vi "REPORT_GEAR_rows_style_pdf.vi"(11 "REPORT_GEAR_all_info":T1) -> (3 "Row  [ ]":T4)   [LabVIEW 2020]
uses:
  <vilib>/Exaprom PDF/Controls/Table Controls/Table Appearance and Font Row [ ].ctl
  <vilib>/Exaprom PDF/Controls/Table Controls/One Row Appearance.ctl
  <vilib>/Exaprom PDF/Controls/Table Controls/Row from to.ctl
  <vilib>/Exaprom PDF/Controls/Table Controls/Cell, Alignment, LS and Font - hide Vmerge.ctl
  <vilib>/Exaprom PDF/Controls/Table Controls/Cell Type, Alignment and LS.ctl
  <vilib>/Exaprom PDF/Controls/Table Controls/Cell Alignment 20px.ctl
  <vilib>/Exaprom PDF/Controls/Table Controls/Text vertical arrangement.ctl
  <vilib>/Exaprom PDF/Controls/Text Controls/Line spacing.ctl
  <vilib>/Exaprom PDF/Controls/Table Controls/Cell Appearance.ctl
  <vilib>/Exaprom PDF/Controls/Table Controls/Cell Border 20 px.ctl
  <vilib>/Exaprom PDF/Controls/Table Controls/Merge Horizontal.ctl
  <vilib>/Exaprom PDF/Controls/Table Controls/Merge Vertical.ctl
  <vilib>/Exaprom PDF/Controls/Font Controls/Font complete cluster.ctl
  <vilib>/Exaprom PDF/Controls/Font Controls/Font size.ctl
  <vilib>/Exaprom PDF/Controls/Font Controls/Font color.ctl
  <vilib>/Exaprom PDF/Controls/Font Controls/Type and encoding.ctl
  <vilib>/Exaprom PDF/Controls/Text Controls/Unicode/Type and run direction.ctl
  typedef/REPORT_GEAR_all_info.ctl
  typedef/REPORT_GEAR_header_data_display.ctl
  typedef/REPORT_GEAR_statuses.ctl
panel:
  # "GEAR INFO SUMMARY"
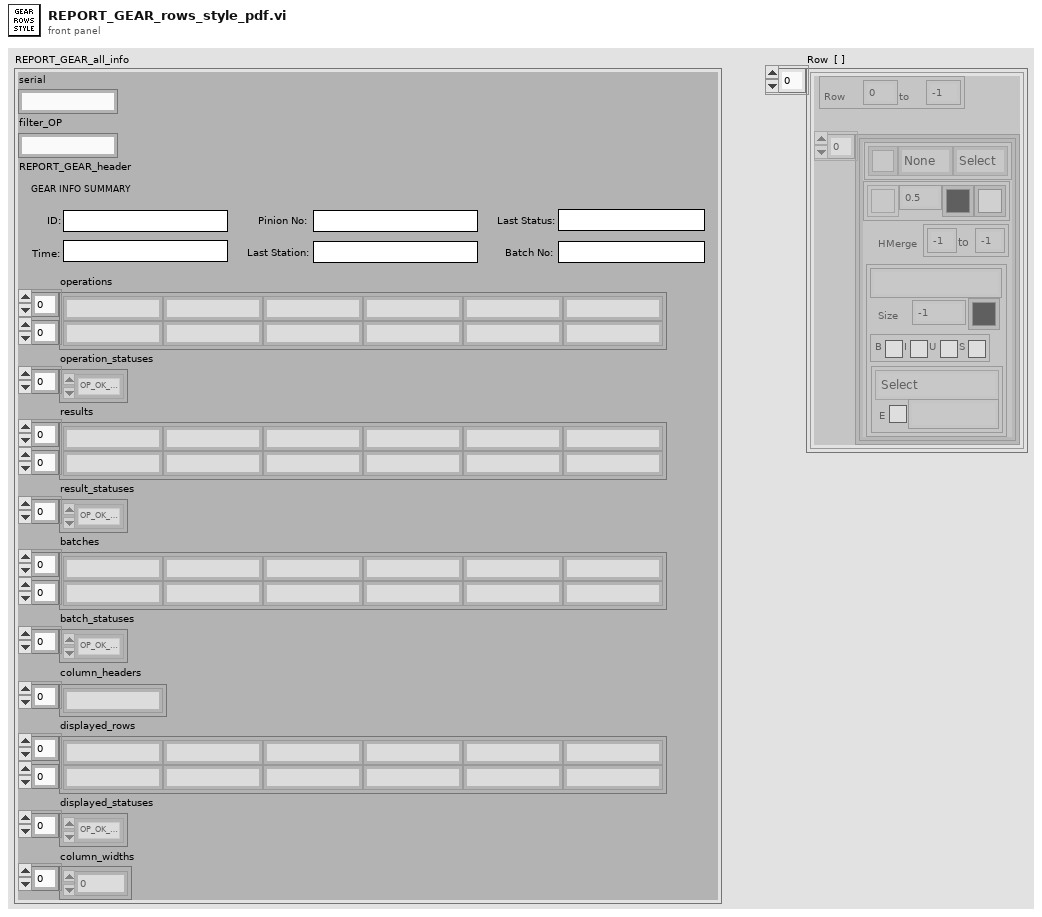
[diagram p1: front panel]
types:
  T1 = typedef "REPORT_GEAR_all_info.ctl" = cluster{"serial":string, "filter_OP":string, "REPORT_GEAR_header":T2, "operations":string[][], "operation_statuses":T3[], "results":string[][], "result_statuses":T3[], "batches":string[][], "batch_statuses":T3[], "column_headers":string[], "displayed_rows":string[][], "displayed_statuses":T3[], "column_widths":i16[]}
  T2 = typedef "REPORT_GEAR_header_data_display.ctl" = cluster{"ID":string, "creation_time":string, "last_station":string, "last_status":string, "pinion_serial":string, "batch_code":string}
  T3 = typedef "REPORT_GEAR_statuses.ctl" = enum16{"OP_OK_hide", "OP_OK_show", "OP_NOK_hide", "OP_NOK_show", "OP_interrupted_hide", "OP_interrupted_show", "OP_in_operation_hide", "OP_in_operation_show", "OP_unexpected_hide", "OP_unexpected_show", "RE_REAL_OK", "RE_REAL_NOK", "RE_STRING", "RE_sub_header", "RE_no_data", "RE_unexpected", "BA_sub_header", "BA_data", "BA_no_data", "AUDIT_RESULT_OK", "AUDIT_RESULT_NOK", "AUDIT_RESULT_UNEXPECTED"}
  T4 = typedef "Table Appearance and Font Row [ ].ctl" = T5[]
  T5 = typedef "One Row Appearance.ctl" = cluster{"Row":T6, "Cell [ ]":T7[]}
  T6 = typedef "Row from to.ctl" = cluster{"From #":i16, "to #":i16}
  T7 = typedef "Cell, Alignment, LS and Font - hide Vmerge.ctl" = cluster{"Text":T8, "Cell Appearance":T12, "HMerge":T14, "VMerge":T15, "Font":T16}
  T8 = typedef "Cell Type, Alignment and LS.ctl" = cluster{"Cell Alignment":T9, "Text rotation":T10, "Line spacing":T11}
  T9 = typedef "Cell Alignment 20px.ctl" = u16
  T10 = typedef "Text vertical arrangement.ctl" = enum16{"None", "Clockwise", "Counterclockwise"}
  T11 = typedef "Line spacing.ctl" = enum16{"Select", "1.0", "1.5", "2.0"}
  T12 = typedef "Cell Appearance.ctl" = cluster{"Border":T13, "Thickness":sgl, "Color":u32, "BG":u32}
  T13 = typedef "Cell Border 20 px.ctl" = u16
  T14 = typedef "Merge Horizontal.ctl" = cluster{"From":i8, "to":i8}
  T15 = typedef "Merge Vertical.ctl" = cluster{"From":i8, "to":i8}
  T16 = typedef "Font complete cluster.ctl" = cluster{"Name":string, "Size":T17, "Color":T18, "Style":cluster{"Bold":bool, "Italic":bool, "Underline":bool, "Strikeout":bool}, "Type":T19}
  T17 = typedef "Font size.ctl" = sgl
  T18 = typedef "Font color.ctl" = u32
  T19 = typedef "Type and encoding.ctl" = cluster{"Type&direction":T20, "Embedded":bool, "Encoding":string}
  T20 = typedef "Type and run direction.ctl" = enum16{"Select", "ASCII", "UTF-16", "UTF-16 (default)", "UTF-16 (LTR)", "UTF-16 (RTL)"}
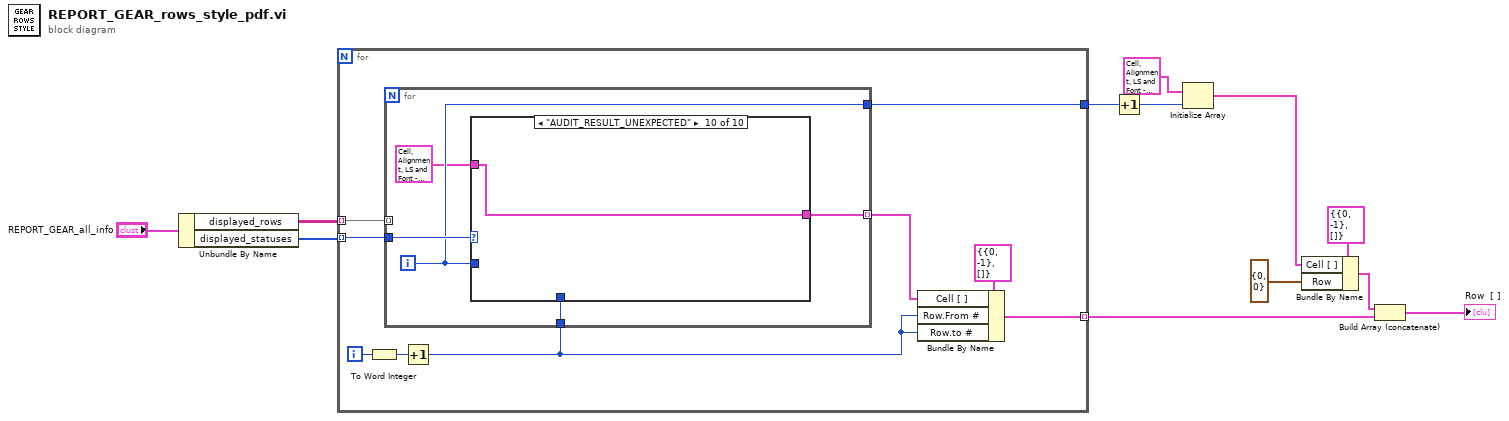
[diagram p0: block diagram]
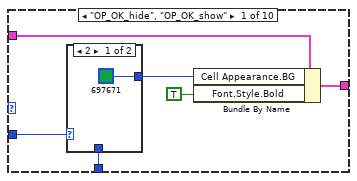
[diagram p2: hidden frame]
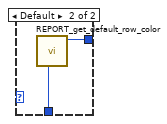
[diagram p3: hidden frame]
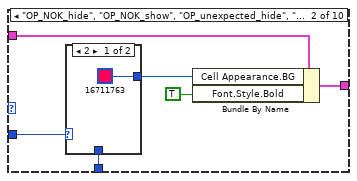
[diagram p4: hidden frame]
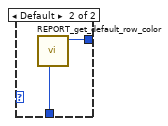
[diagram p5: hidden frame]
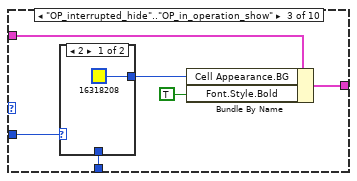
[diagram p6: hidden frame]
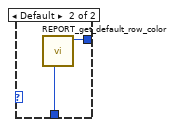
[diagram p7: hidden frame]
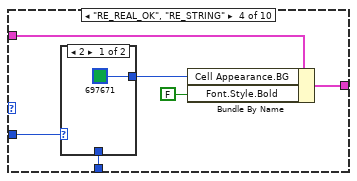
[diagram p8: hidden frame]
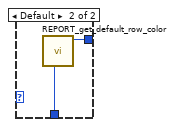
[diagram p9: hidden frame]
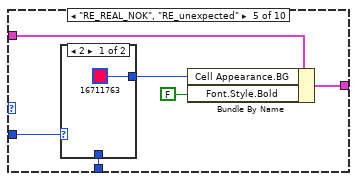
[diagram p10: hidden frame]
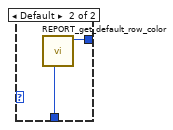
[diagram p11: hidden frame]
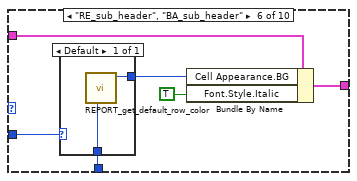
[diagram p12: hidden frame]
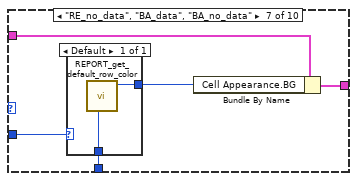
[diagram p13: hidden frame]
diagram:
  n1 = Unbundle By Name("REPORT_GEAR_all_info") -> ("displayed_rows"=w11:string[][], "displayed_statuses"=w10:T3[])
  n2 = for {
    tunnel: w11 -> [w17] mode=indexing
    tunnel: w10 -> [w16] mode=indexing
    tunnel: [w20] -> w8 mode=indexing
    tunnel: [w13] -> w2
    i -> [w19]
    n3 = To Word Integer(number=w19) -> (16bit integer=w18:i16)
    n4 = Increment(x=w18) -> (x+1=w14:i16)
    n5 = for {
      tunnel: w17 -> [_] mode=indexing
      tunnel: w16 -> [w26]
      tunnel: [w25] -> w15 mode=indexing
      tunnel: w14 -> [w24]
      tunnel: [w23] -> w13
      i -> [w23]
      n6 = case shown="\"AUDIT_RESULT_UNEXPECTED\"" w26 {
        tunnel: T7 {"Text"={"Cell Alignment"=0, "Text rotation"=enum."None", "Line spacing"=enum."Select"}, "Cell Appearance"={"Border"=5, "Thickness"=0.5, "Color"=0, "BG"=16448250}, "HMerge"={"From"=-1, "to"=-1}, "VMerge"={"From"=-1, "to"=-1}, "Font"={"Name"="Consolas", "Size"=10.0, "Color"=0, "Style"={"Bold"=FALSE, "Italic"=FALSE, "Underline"=FALSE, "Strikeout"=FALSE}, "Type"={"Type&direction"=enum."ASCII", "Embedded"=FALSE, "Encoding"="CP855"}}} ("Cell, Alignment, LS and Font") -> [w32 w39 w48 w57 w66 w75 w83 w87 w88 w89]
        tunnel: [w29 w38 w47 w56 w65 w74 w81 w87 w88 w89] -> w25
        tunnel: w23 -> [w28 w37 w46 w55 w64 w73 w82 _ _ _]
        tunnel: w24 -> [w27 w36 w45 w54 w63 w72 w80 _ _ _]
        frame "OP_OK_hide", "OP_OK_show" {
          n7 = case shown="2" w28 {
            tunnel: [u32 697671 w35] -> w30
            tunnel: w27 -> [_ w34]
            frame 2 {
            }
            frame Default {
              n8 = call "REPORT_get_default_row_color.vi"("row"=w34) -> ("color"=w35:u32)  [unwired: 10 in]
            }
          }
          n9 = Bundle By Name(cluster=w32, "Cell Appearance.BG"=w30, "Font.Style.Bold"=TRUE ("Active Cell:Cell Font:Bold")) -> (w29:T7)
        }
        frame "OP_NOK_hide", "OP_NOK_show", "OP_unexpected_hide", "OP_unexpected_show" {
          n10 = case shown="2" w37 {
            tunnel: [u32 16711763 w44] -> w40
            tunnel: w36 -> [_ w43]
            frame 2 {
            }
            frame Default {
              n11 = call "REPORT_get_default_row_color.vi"("row"=w43) -> ("color"=w44:u32)  [unwired: 10 in]
            }
          }
          n12 = Bundle By Name(cluster=w39, "Cell Appearance.BG"=w40, "Font.Style.Bold"=TRUE ("Active Cell:Cell Font:Bold")) -> (w38:T7)
        }
        frame "OP_interrupted_hide".."OP_in_operation_show" {
          n13 = case shown="2" w46 {
            tunnel: [u32 16318208 w53] -> w49
            tunnel: w45 -> [_ w52]
            frame 2 {
            }
            frame Default {
              n14 = call "REPORT_get_default_row_color.vi"("row"=w52) -> ("color"=w53:u32)  [unwired: 10 in]
            }
          }
          n15 = Bundle By Name(cluster=w48, "Cell Appearance.BG"=w49, "Font.Style.Bold"=TRUE ("Active Cell:Cell Font:Bold")) -> (w47:T7)
        }
        frame "RE_REAL_OK", "RE_STRING" {
          n16 = case shown="2" w55 {
            tunnel: [u32 697671 w62] -> w58
            tunnel: w54 -> [_ w61]
            frame 2 {
            }
            frame Default {
              n17 = call "REPORT_get_default_row_color.vi"("row"=w61) -> ("color"=w62:u32)  [unwired: 10 in]
            }
          }
          n18 = Bundle By Name(cluster=w57, "Cell Appearance.BG"=w58, "Font.Style.Bold"=FALSE ("Active Cell:Cell Font:Bold")) -> (w56:T7)
        }
        frame "RE_REAL_NOK", "RE_unexpected" {
          n19 = case shown="2" w64 {
            tunnel: [u32 16711763 w71] -> w67
            tunnel: w63 -> [_ w70]
            frame 2 {
            }
            frame Default {
              n20 = call "REPORT_get_default_row_color.vi"("row"=w70) -> ("color"=w71:u32)  [unwired: 10 in]
            }
          }
          n21 = Bundle By Name(cluster=w66, "Cell Appearance.BG"=w67, "Font.Style.Bold"=FALSE ("Active Cell:Cell Font:Bold")) -> (w65:T7)
        }
        frame "RE_sub_header", "BA_sub_header" {
          n22 = case shown="Default" w73 {
            tunnel: [w79] -> w76
            tunnel: w72 -> [w78]
            frame Default {
              n23 = call "REPORT_get_default_row_color.vi"("row"=w78) -> ("color"=w79:u32)  [unwired: 10 in]
            }
          }
          n24 = Bundle By Name(cluster=w75, "Cell Appearance.BG"=w76, "Font.Style.Italic"=TRUE ("Active Cell:Cell Font:Bold")) -> (w74:T7)
        }
        frame "RE_no_data", "BA_data", "BA_no_data" {
          n25 = case shown="Default" w82 {
            tunnel: [w86] -> w84
            tunnel: w80 -> [w85]
            frame Default {
              n26 = call "REPORT_get_default_row_color.vi"("row"=w85) -> ("color"=w86:u32)  [unwired: 10 in]
            }
          }
          n27 = Bundle By Name(cluster=w83, "Cell Appearance.BG"=w84) -> (w81:T7)
        }
        frame "AUDIT_RESULT_OK" {
        }
        frame "AUDIT_RESULT_NOK" {
        }
        frame "AUDIT_RESULT_UNEXPECTED" {
        }
      }
    }
    n28 = Bundle By Name(cluster=T5 {"Row"={"From #"=0, "to #"=-1}, "Cell [ ]"=[]} ("Row Appearance and Font  [ ]"), "Cell [ ]"=w15, "Row.From #"=w14, "Row.to #"=w14) -> (w20:T5)
  }
  n29 = Increment(x=w2) -> (x+1=w1:i32)
  n30 = Initialize Array(T7 {"Text"={"Cell Alignment"=0, "Text rotation"=enum."None", "Line spacing"=enum."Select"}, "Cell Appearance"={"Border"=5, "Thickness"=1.5, "Color"=16777228, "BG"=16448250}, "HMerge"={"From"=-1, "to"=-1}, "VMerge"={"From"=-1, "to"=-1}, "Font"={"Name"="Consolas", "Size"=10.0, "Color"=16777228, "Style"={"Bold"=TRUE, "Italic"=FALSE, "Underline"=FALSE, "Strikeout"=FALSE}, "Type"={"Type&direction"=enum."ASCII", "Embedded"=FALSE, "Encoding"="CP855"}}} ("Cell, Alignment, LS and Font"), w1) -> (w4:T7[])
  n31 = Bundle By Name(cluster=T5 {"Row"={"From #"=0, "to #"=-1}, "Cell [ ]"=[]} ("Row Appearance and Font  [ ]"), "Cell [ ]"=w4, "Row"=T6 {"From #"=0, "to #"=0}) -> (w6:T5)
  n32 = Build Array (concatenate)(w6, w8) -> (→"Row  [ ]":T5[])
